vi "PI_valvula3.vi"(9 "controlON":bool, 10 "Temperatura":dbl format="%.2f", 11 "Setpoint T":dbl) -> (3 "PWM (%)":dbl)   [LabVIEW 2021, in "DAQ_Termopares.lvlib"]
uses:
  DAQ/DAQ_Termopares.lvlib
  <vilib>/addons/control/pid/NI_PID_pid.lvlib
  <vilib>/addons/control/pid/pid.llb/PID (DBL).vi
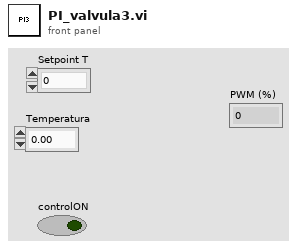
[diagram p1: front panel]
types:
  T1 = cluster{"proportional gain (Kc)":dbl, "integral time (Ti, min)":dbl, "derivative time (Td, min)":dbl}
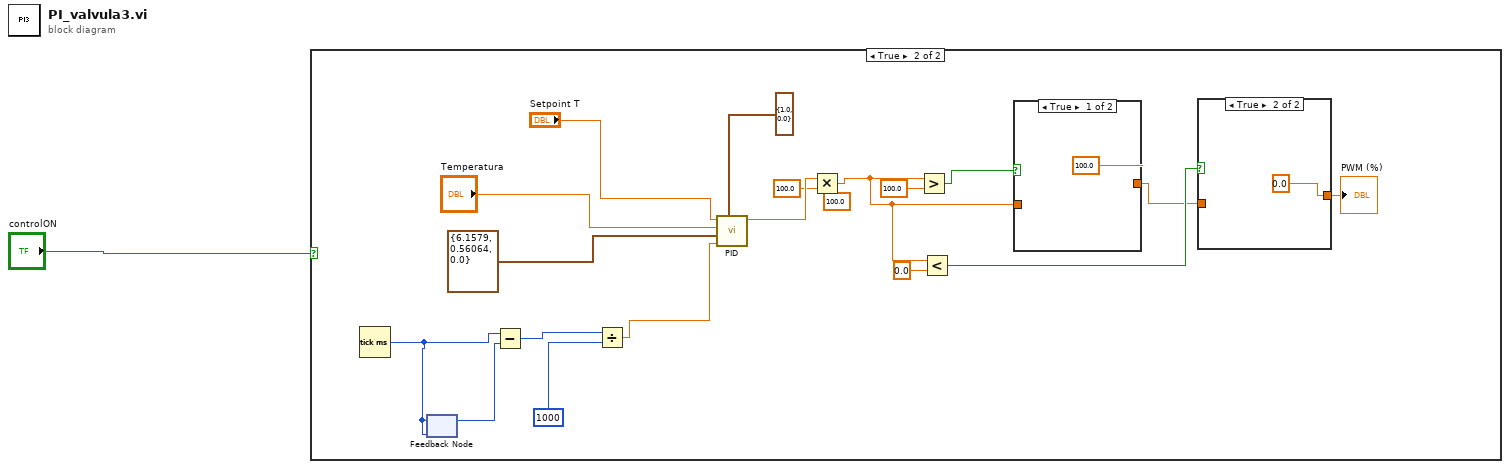
[diagram p0: block diagram]
diagram:
  n1 = case shown="True" "controlON" {
    frame False {
    }
    frame True {
      (unwired) 100.0 ("y")
      n2 = Tick Count (ms)() -> (millisecond timer value=w19:u32)
      n3 = feedback #1(w19) -> (w18:u32)
      n4 = feedback-in #1(w19) -> ()
      n5 = Subtract(x=w19, y=w18) -> (x-y=w16:u32)
      n6 = Divide(x=w16, y=1000) -> (x/y=w5:dbl)
      n7 = call-poly <vilib>:"PID.vi"("output range"=cluster{"output high":dbl, "output low":dbl} {"output high"=1.0, "output low"=0.0}, "dt (s)"=w5, "PID gains"=T1 {"proportional gain (Kc)"=6.1579, "integral time (Ti, min)"=0.56064, "derivative time (Td, min)"=0.0}, "process variable"="Temperatura", "setpoint"="Setpoint T") -> ("output"=w13:dbl)  [unwired: 5 in, 1 out]
      n8 = Multiply(x=w13, y=100.0) -> (x*y=w8:dbl)
      n9 = Greater?(x=w8, y=100.0) -> (0:w9:bool)
      n10 = Less?(x=w8, y=0.0) -> (x < y?=w7:bool)
      n11 = case shown="True" w9 {
        tunnel: w8 -> [_ w23]
        tunnel: [100.0 w23] -> w6
        frame True {
        }
        frame False {
        }
      }
      n12 = case shown="True" w7 {
        tunnel: w6 -> [w20 _]
        tunnel: [w20 0.0] -> w2
        frame False {
        }
        frame True {
        }
      }
      "PWM (%)" <- w2
    }
  }
